vi "Get Sender.vi"(11 "Setup Msg Strategy in":refnum<class "Setup Msg Strategy.lvclass">) -> (2 "Sender":refnum<class "Sender.lvclass">)   [LabVIEW 2021, in "jettl.lvlib" / "Setup Msg Strategy.lvlib" / "Setup Msg Strategy.lvclass"]
uses:
  Setup Msg Strategy.lvclass
  Setup Msg Strategy.lvclass/Setup Msg Strategy.ctl
  Sender/Sender/Sender.lvclass
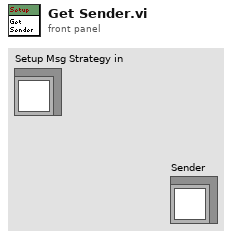
[diagram p1: front panel]
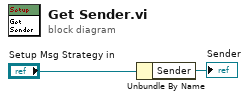
[diagram p0: block diagram]
diagram:
  n1 = Unbundle By Name("Setup Msg Strategy in") -> ("Sender"=→"Sender":refnum<class "Sender.lvclass">)
